vi "prime_factorization.vi"() -> ()   [LabVIEW 2021]
panel:
  out "found":bool
  out "b":i32
  out "a":u32
  in  "n":u32
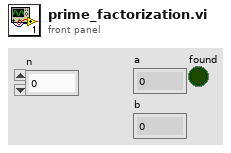
[diagram p1: front panel]
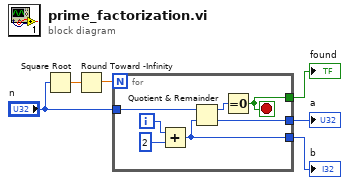
[diagram p0: block diagram]
diagram:
  n1 = Square Root(x="n") -> (sqrt(x)=w6:dbl)
  n2 = Round Toward -Infinity(1:w6) -> (0:w5:dbl)
  n3 = for {
    N: w5 -> [_]
    tunnel: "n" -> [w11]
    tunnel: [w9] -> w3
    tunnel: [w8] -> w2
    tunnel: [w7] -> w1
    i -> [w13]
    stop <- w7 stop-if-true
    n4 = Add(x=w13, y=2) -> (x+y=w8:i32)
    n5 = Quotient & Remainder(x=w11, y=w8) -> (x-y*floor(x/y)=w10:u32, floor(x/y)=w9:u32)
    n6 = Equal To 0?(x=w10) -> (x = 0?=w7:bool)
  }
  "a" <- w3
  "b" <- w2
  "found" <- w1
